vi "Subsystem 3.vi"() -> ()   [LabVIEW 2014]
uses:
  <vilib>/myRIO/Instrument Drivers/Onboard IO/DIO/typedefs/DIO Reference.ctl
  <vilib>/myRIO/Common/Instrument Driver Framework/Utilities/typedefs/myRIO Generic Hardware Reference.ctl
  <vilib>/myRIO/Common/Instrument Driver Framework/Utilities/typedefs/Hardware Version Enum.ctl
  <vilib>/myRIO/Common/Instrument Driver Framework/Utilities/typedefs/myRIO v1.0 Reference.ctl
  <vilib>/myRIO/Common/Instrument Driver Framework/Utilities/typedefs/Generic FPGA Reference.ctl
  <vilib>/myRIO/Common/Instrument Driver Framework/myRIO v1.0/DIO/typedefs/DIO Channels List.ctl
  <vilib>/myRIO/Common/Instrument Driver Framework/myRIO v1.0/DIO/typedefs/DIO Channels Enum.ctl
  <vilib>/userdefined/High Color/nirio_resource_hc.ctl
  <vilib>/myRIO/Instrument Drivers/Onboard IO/PWM/typedefs/PWM Reference.ctl
  <vilib>/myRIO/Common/Instrument Driver Framework/myRIO v1.0/PWM/typedefs/PWM Channels Enum.ctl
  <vilib>/myRIO/Instrument Drivers/Onboard IO/PWM/typedefs/PWM Configuration.ctl
  <vilib>/myRIO/Common/Instrument Driver Framework/Utilities/vis/Is FPGA Ref Available.vi
  <vilib>/myRIO/Common/Instrument Driver Framework/myRIO v1.0/PWM/vis/myRIO v1.1 Open PWM.vi
  <vilib>/myRIO/Instrument Drivers/Onboard IO/PWM/vis/Set Duty Cycle and Frequency.vi
  <vilib>/myRIO/Common/Instrument Driver Framework/myRIO v1.0/DIO/vis/myRIO v1.1 Open DIO.vi
  <vilib>/myRIO/Instrument Drivers/Onboard IO/DIO/vis/Read.vi
  <vilib>/myRIO/Instrument Drivers/Onboard IO/DIO/vis/Write.vi
  <vilib>/myRIO/Common/Instrument Driver Framework/Utilities/vis/Validate Channels.vi
  <vilib>/myRIO/Common/Instrument Driver Framework/myRIO v1.0/PWM/vis/myRIO v1.0 Reserve PWM.vi
  <vilib>/myRIO/Common/Instrument Driver Framework/myRIO v1.0/DIO/vis/myRIO v1.0 Reserve DIO.vi
  <vilib>/myRIO/Common/Instrument Driver Framework/myRIO v1.0/UART/vis/myRIO v1.0 Close UART.vi
  <vilib>/myRIO/Common/Instrument Driver Framework/myRIO v1.0/PWM/vis/myRIO v1.0 Build MUX Configuration PWM.vi
  <vilib>/myRIO/Common/Instrument Driver Framework/myRIO v1.0/Resource Manager/vis/myRIO v1.0 Reserve Channel List.vi
  <vilib>/myRIO/Common/Instrument Driver Framework/myRIO v1.0/DIO/vis/myRIO v1.0 Build MUX Configuration DIO.vi
  <vilib>/myRIO/Common/Instrument Driver Framework/myRIO v1.0/Resource Manager/vis/myRIO v1.0 Create Configuration List.vi
  <vilib>/myRIO/Common/Instrument Driver Framework/myRIO v1.0/Resource Manager/vis/myRIO v1.0 Reserve Channel.vi
  <vilib>/myRIO/Common/Instrument Driver Framework/myRIO v1.0/Resource Manager/vis/myRIO v1.0 Unreserve Channel.vi
  <vilib>/myRIO/Common/Instrument Driver Framework/myRIO v1.0/Resource Manager/vis/myRIO v1.0 Build Mutex Name.vi
  <vilib>/Utility/VariantDataType/GetNumericInfo.vi
  <vilib>/Utility/error.llb/Error Cluster From Error Code.vi
  <vilib>/myRIO/Common/Instrument Driver Framework/myRIO v1.0/myRIO v1.1 Open.vi
  <vilib>/myRIO/Common/Instrument Driver Framework/Utilities/vis/IO Manager.vi
  <vilib>/myRIO/Common/Instrument Driver Framework/Utilities/vis/Configuration Manager.vi
  <vilib>/myRIO/Common/Instrument Driver Framework/myRIO v1.0/Resource Manager/vis/myRIO v1.0 Configure IO.vi
  <vilib>/myRIO/Common/Instrument Driver Framework/myRIO v1.0/myRIO v1.0 Close.vi
  <vilib>/myRIO/Common/Instrument Driver Framework/myRIO v1.0/DIO/vis/myRIO v1.0 Read DIO.vi
  <vilib>/functionblocks/Edge Detection/One Shot Falling With Input/One Shot Falling With Input.vi
  <vilib>/myRIO/Common/Instrument Driver Framework/myRIO v1.0/PWM/vis/myRIO v1.0 Write PWM.vi
  <vilib>/myRIO/Common/Instrument Driver Framework/myRIO v1.0/DIO/vis/myRIO v1.0 Write DIO.vi
  <vilib>/myRIO/Common/Instrument Driver Framework/Utilities/vis/FPGA Ref Manager.vi
  <vilib>/myRIO/Common/Instrument Driver Framework/myRIO v1.0/myRIO v1.0 Reset FPGA.vi
  <vilib>/myRIO/Common/Instrument Driver Framework/myRIO v1.0/IRQ/vis/myRIO v1.0 IRQ Info FGV.vi
  <vilib>/myRIO/Common/Instrument Driver Framework/myRIO v1.0/IRQ/vis/myRIO v1.0 Timer IRQ Info FGV.vi
  <vilib>/myRIO/Common/Instrument Driver Framework/myRIO v1.0/IRQ/vis/myRIO v1.0 ISR Agent.vi
  <vilib>/myRIO/Express VI/Onboard IO/DI/DI Express VI.xnode
  <vilib>/myRIO/Instrument Drivers/Onboard IO/DIO/vis/myRIO DIO Open.xnode
  <vilib>/functionblocks/FB Core/FB Core.xnode
  <vilib>/myRIO/Express VI/Onboard IO/PWM/PWM Express VI.xnode
  <vilib>/myRIO/Instrument Drivers/Onboard IO/PWM/vis/myRIO PWM Open.xnode
  <vilib>/myRIO/Express VI/Onboard IO/DO/DO Express VI.xnode
  <vilib>/myRIO/Express VI/Onboard Devices/LED/LED Express VI.xnode
  <vilib>/myRIO/Instrument Drivers/Utilities/Utilities.lvlib
  <vilib>/myRIO/Instrument Drivers/Onboard IO/DIO/DIO.lvlib
  <vilib>/functionblocks/NI_FunctionBlock Libraries.lvlib
  <vilib>/myRIO/Instrument Drivers/Onboard IO/PWM/PWM.lvlib
panel:
  in  "stop":bool
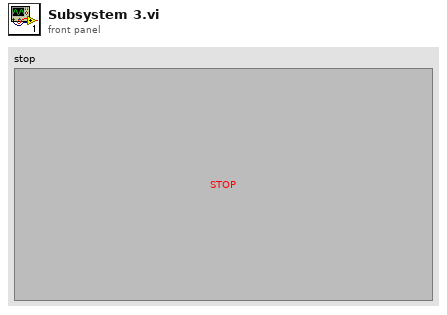
[diagram p1: front panel]
types:
  T1 = typedef "PWM.lvlib/PWM Reference.ctl" = cluster{"myRIO Reference":T2, "PWM Channels Enum":T6, "PWM Configuration":T7}
  T2 = typedef "myRIO Generic Hardware Reference.ctl" = cluster{"myRIO Model":T3, "myRIO Hardware Reference":T4}
  T3 = typedef "Hardware Version Enum.ctl" = enum16{"Unknown", "myRIO-1900", "myRIO-1950"}
  T4 = typedef "myRIO v1.0 Reference.ctl" = cluster{"Generic FPGA Reference":T5, "Allow multiple opens":bool}
  T5 = typedef "Generic FPGA Reference.ctl" = refnum<k20>
  T6 = typedef "PWM Channels Enum.ctl" = enum16{"Not Connected", "C/PWM0", "C/PWM1", "A/PWM0", "A/PWM1", "A/PWM2", "B/PWM0", "B/PWM1", "B/PWM2"}
  T7 = typedef "PWM.lvlib/PWM Configuration.ctl" = cluster{"Frequency":dbl, "Duty Cycle":dbl}
  T8 = typedef "nirio_resource_hc.ctl" = tag
  T9 = typedef "DIO.lvlib/DIO Reference.ctl" = cluster{"myRIO Reference":T2, "DIO Channels List":T10}
  T10 = typedef "DIO Channels List.ctl" = T11[]
  T11 = typedef "DIO Channels Enum.ctl" = enum16{"Not Connected", "C/DIO0", "C/DIO1", "C/DIO2", "C/DIO3", "C/DIO4", "C/DIO5", "C/DIO6", "C/DIO7", "A/DIO0", "A/DIO1", "A/DIO2", "A/DIO3", "A/DIO4", "A/DIO5", "A/DIO6", "A/DIO7", "A/DIO8", "A/DIO9", "A/DIO10", "A/DIO11", "A/DIO12", "A/DIO13", "A/DIO14", "A/DIO15", "B/DIO0", "B/DIO1", "B/DIO2", "B/DIO3", "B/DIO4", "B/DIO5", "B/DIO6", "B/DIO7", "B/DIO8", "B/DIO9", "B/DIO10", "B/DIO11", "B/DIO12", "B/DIO13", "B/DIO14", "B/DIO15", "LED0", "LED1", "LED2", "LED3", "Button0"}
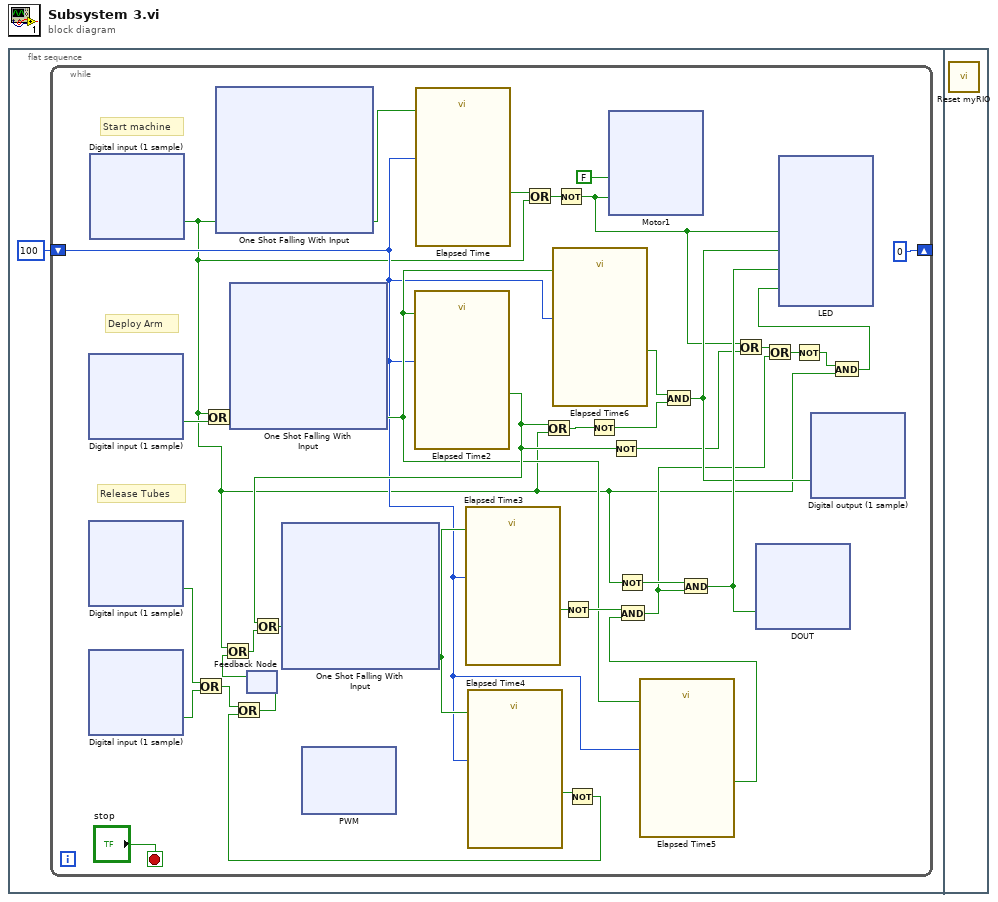
[diagram p0: block diagram]
diagram:
  n1 = flat-sequence {
    frame #0 {
      n2 = while {
        shift-right: [0] -> _
        shift-left: 100 -> [w11]
        stop <- "stop" stop-if-true
        # "Release Tubes"
        # "Deploy Arm"
        # "Start machine"
        n3 = xnode "Digital input (1 sample)"() -> ("B/DIO2 (Pin 15)"=w35:bool)  [unwired: 1 in, 1 out]
        n4 = xnode "Digital input (1 sample)"() -> ("B/DIO1 (Pin 13)"=w34:bool)  [unwired: 1 in, 1 out]
        n5 = xnode "Digital input (1 sample)"() -> ("B/DIO0 (Pin 11)"=w30:bool)  [unwired: 1 in, 1 out]
        n6 = xnode "Digital input (1 sample)"() -> ("B/DIO5 (Pin 21)"=w2:bool)  [unwired: 1 in, 1 out]
        n7 = Or(x=w34, y=w30) -> (x .or. y?=w32:bool)
        n8 = Or(x=w2, y=w35) -> (x .or. y?=w27:bool)
        n9 = xnode "One Shot Falling With Input"("input"=w2) -> ("output"=w28:bool)  [unwired: 1 in, 1 out]
        n10 = xnode "One Shot Falling With Input"("input"=w27) -> ("output"=w12:bool)  [unwired: 1 in, 1 out]
        n11 = feedback #1() -> (w13:bool)  [unwired: 1 in]
        n12 = Or(x=w2, y=w13) -> (x .or. y?=w14:bool)
        n13 = xnode "PWM"() -> ()  [unwired: 1 in, 1 out]
        n14 = call "Elapsed Time2"("Reset"=w12, "Set Start Time (s)"=w11) -> ("Time has Elapsed"=w15:bool)  [unwired: 10 in, 7 out]
        n15 = Or(x=w15, y=w14) -> (x .or. y?=w24:bool)
        n16 = xnode "One Shot Falling With Input"("input"=w24) -> ("output"=w26:bool)  [unwired: 1 in, 1 out]
        n17 = call "Elapsed Time"("Reset"=w28, "Set Start Time (s)"=w11) -> ("Time has Elapsed"=w7:bool)  [unwired: 10 in, 7 out]
        n18 = call "Elapsed Time3"("Reset"=w26, "Set Start Time (s)"=w11) -> ("Time has Elapsed"=w36:bool)  [unwired: 10 in, 7 out]
        n19 = call "Elapsed Time4"("Reset"=w26, "Set Start Time (s)"=w11) -> ("Time has Elapsed"=w33:bool)  [unwired: 10 in, 7 out]
        n20 = Or(x=w7, y=w2) -> (x .or. y?=w16:bool)
        n21 = Or(x=w15, y=w2) -> (x .or. y?=w17:bool)
        n22 = call "Elapsed Time6"("Reset"=w12, "Set Start Time (s)"=w11) -> ("Time has Elapsed"=w8:bool)  [unwired: 10 in, 7 out]
        n23 = Not(x=w16) -> (.not. x?=w5:bool)
        n24 = Not(x=w36) -> (.not. x?=w29:bool)
        n25 = Not(x=w33) -> (.not. x?=w6:bool)
        n26 = Or(x=w32, y=w6) -> (x .or. y?=w31:bool)
        n27 = feedback-in #1(w31) -> ()
        n28 = Not(x=w17) -> (.not. x?=w9:bool)
        n29 = xnode "Motor1"("A/DIO6 (Pin 23)"=FALSE, "A/DIO7 (Pin 25)"=w5) -> ()  [unwired: 1 in, 1 out]
        n30 = Not(x=w15) -> (.not. x?=w3:bool)
        n31 = Not(x=w2) -> (.not. x?=w18:bool)
        n32 = call "Elapsed Time5"("Reset"=w12, "Set Start Time (s)"=w11) -> ("Time has Elapsed"=w25:bool)  [unwired: 10 in, 7 out]
        n33 = And(x=w29, y=w25) -> (x .and. y?=w4:bool)
        n34 = And(x=w8, y=w9) -> (x .and. y?=w10:bool)
        n35 = And(x=w18, y=w4) -> (x .and. y?=w19:bool)
        n36 = Or(x=w5, y=w3) -> (x .or. y?=w21:bool)
        n37 = xnode "DOUT"("A/DIO3 (Pin 17)"=w19) -> ()  [unwired: 1 in, 1 out]
        n38 = Or(x=w21, y=w4) -> (x .or. y?=w20:bool)
        n39 = Not(x=w20) -> (.not. x?=w23:bool)
        n40 = xnode "Digital output (1 sample)"("A/DIO2 (Pin 15)"=w10) -> ()  [unwired: 1 in, 1 out]
        n41 = And(x=w23, y=w2) -> (x .and. y?=w22:bool)
        n42 = xnode "LED"("Motor"=w5, "Arm"=w10, "Tube"=w19, "Ready"=w22) -> ()  [unwired: 1 in, 1 out]
      }
    }
    frame #1 {
      n43 = call <vilib>:"Reset myRIO.vi"() -> ()  [unwired: 11 in, 1 out]
    }
  }
